vi "Query Instrument Identifier.vi"(0 "VISA resource name":refnum<visa-resource-name>, 5 "Logical Instrument Name":string, 11 "error in (no error)":errorcluster) -> (4 "VISA resource name out":refnum<visa-resource-name>, 6 "Logical Instrument Number":u32 max=12 step=1, 15 "error out":errorcluster)   [LabVIEW 2020, in "NH Research Regenerative Test Series.lvlib"]
doc: "Returns the <B>Logical Instrument Number</B> for the input <B>Logical Instrument Name</B>.\n\nNOTE: The 4900 only has one logical instrument so the only valid instrument number is 1."
uses:
  NH Research Regenerative Test Series.lvlib
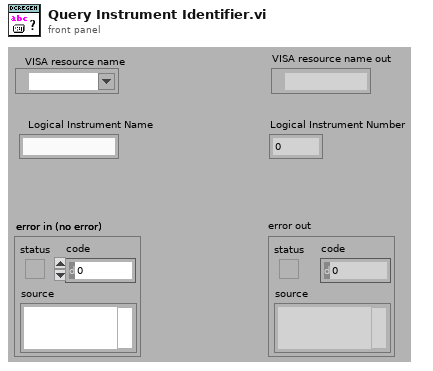
[diagram p1: front panel]
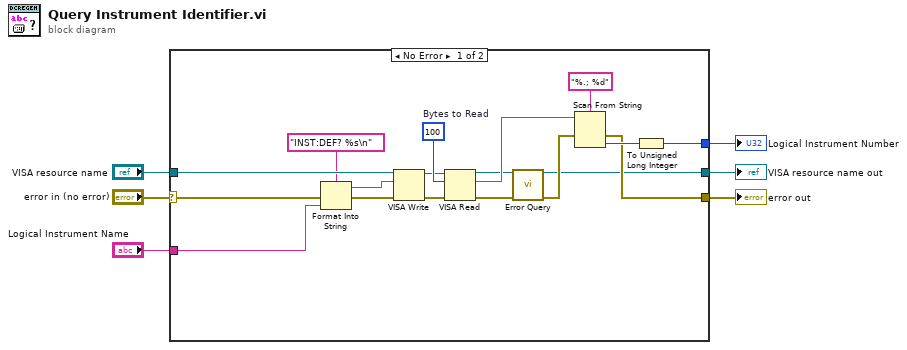
[diagram p0: block diagram]
diagram:
  n1 = case shown="No Error" "error in (no error)" {
    selector: "error in (no error)" -> [w21 w26]
    tunnel: "VISA resource name" -> [w24 w25]
    tunnel: [w8 w25] -> w5
    tunnel: [w9 w26] -> w4
    tunnel: "Logical Instrument Name" -> [w19 _]
    tunnel: [w7 _] -> w1
    frame No Error {
      w18 = u32 100  # Bytes to Read
      n2 = Format Into String(format string="INST:DEF? %s\n" ("Command"), error in=w21, w19) -> (resulting string=w22:string, error out=w20:errorcluster)  [unwired: 1 in]
      n3 = VISA Write(VISA resource name=w24, write buffer=w22, error in (no error)=w20) -> (VISA resource name out=w10:refnum<visa-resource-name>, error out=w11:errorcluster)  [unwired: 1 out]
      n4 = VISA Read(VISA resource name=w10, byte count=w18, error in (no error)=w11) -> (VISA resource name out=w15:refnum<visa-resource-name>, read buffer=w17:string, error out=w14:errorcluster)  [unwired: 1 out]
      n5 = call "Error Query.vi"("VISA resource name"=w15, "error in (no error)"=w14) -> ("VISA resource name out"=w8:refnum<visa-resource-name>, "error out"=w13:errorcluster)  [unwired: 10 in, 2 out]
      n6 = Scan From String(format string="%.; %d", input string=w17, error in=w13) -> (error out=w9:errorcluster, output 1=w12:i32)  [unwired: 2 in, 2 out]
      n7 = To Unsigned Long Integer(number=w12) -> (unsigned 32bit integer=w7:u32)
    }
    frame Error {
    }
  }
  "error out" <- w4
  "VISA resource name out" <- w5
  "Logical Instrument Number" <- w1
